vi "GCF(U64).vi"(10 "B":u64, 11 "A":u64) -> (3 "GCF":u64)   [LabVIEW 2023, in "d8.lvlib"]
uses:
  d8.lvlib
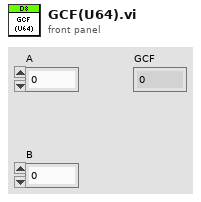
[diagram p1: front panel]
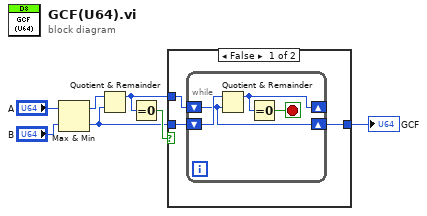
[diagram p0: block diagram]
diagram:
  n1 = Max & Min(x="A", y="B") -> (max(x,y)=w4:u64, min(x,y)=w2:u64)
  n2 = Quotient & Remainder(x=w4, y=w2) -> (x-y*floor(x/y)=w1:u64)  [unwired: 1 out]
  n3 = Equal To 0?(x=w1) -> (x = 0?=w3:bool)
  n4 = case shown="False" w3 {
    tunnel: [w10 w15] -> w7
    tunnel: w2 -> [w9 w15]
    tunnel: w1 -> [w8 _]
    frame False {
      n5 = while {
        shift-right: [w12] -> w10
        shift-left: w9 -> [w13]
        shift-right: [w11] -> _
        shift-left: w8 -> [w12]
        stop <- w14 stop-if-true
        n6 = Quotient & Remainder(x=w13, y=w12) -> (x-y*floor(x/y)=w11:u64)  [unwired: 1 out]
        n7 = Equal To 0?(x=w11) -> (x = 0?=w14:bool)
      }
    }
    frame True {
    }
  }
  "GCF" <- w7
